vi "DO Max no.of Rows.vi"(8 "error in":errorcluster, 10 "Index Array":i32[](array[numeric]), 11 "Message info array":T1[](array[typedef])) -> (0 "error out":errorcluster, 3 "Incremented index":i32[](array[numeric]))   [LabVIEW 2024]
doc: "All Rights Reserved © 2017 SyncSols"
uses:
  Digital Dynamic Cluster.ctl
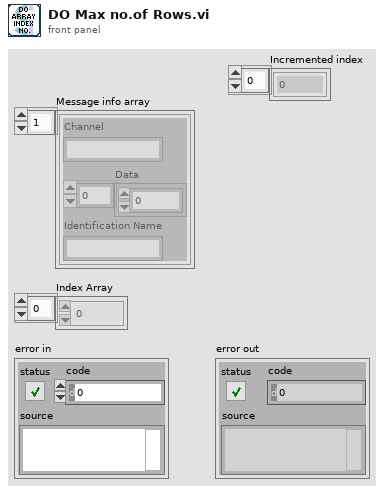
[diagram p1: front panel]
types:
  T1 = typedef "Digital Dynamic Cluster.ctl" = cluster{"Channel":string, "Data":u8[], "Identification Name":string}
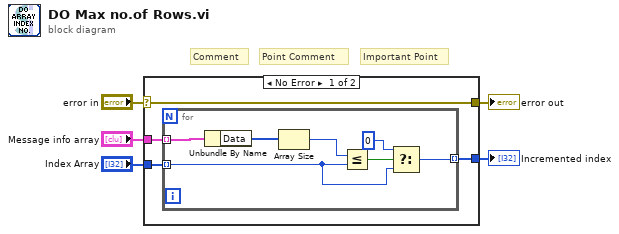
[diagram p0: block diagram]
diagram:
  # "Important Point"
  # "Point Comment"
  # "Comment"
  n1 = case shown="No Error" "error in" {
    selector: "error in" -> [w9 w17]
    tunnel: [w9 w17] -> w5
    tunnel: "Message info array" -> [w8 _]
    tunnel: "Index Array" -> [w7 _]
    tunnel: [w6 _] -> w1
    frame No Error {
      n2 = for {
        tunnel: w8 -> [w16] mode=indexing
        tunnel: w7 -> [w10] mode=indexing
        tunnel: [w11] -> w6 mode=indexing
        n3 = Unbundle By Name(w16) -> ("Data"=w15:u8[])
        n4 = Array Size(array=w15) -> (size(s)=w14:i32)
        n5 = Less Or Equal?(x=w14, y=w10) -> (x <= y?=w13:bool)
        n6 = Select(t=0, s=w13, f=w10) -> (s? t:f=w11:i32)
      }
    }
    frame Error {
    }
  }
  "error out" <- w5
  "Incremented index" <- w1
